vi "ATF-Connect disconnect button logic.vi"(8 "error in":errorcluster, 10 "Select type":T1, 11 "?":T2) -> (0 "error out":errorcluster, 3 "status":string)   [LabVIEW 2022 SP3]
uses:
  Controls/main case.ctl
  Controls/SeCrTs-boolean ref.ctl
  Controls/SeCrTs-EPV .ctl
  Controls/Commands to log.ctl
  UI Message handler/Message Queue/All Message Queues.ctl
  UI Message handler/Message Queue/Message Cluster.ctl
  Controls/SeCrTs-Notifier ctl.ctl
  Controls/SeCrTs-NS Data type.ctl
  Controls/ATF-Select device.ctl
  72e63059-1317-46b0-bf65-451624e866a9.vi
  5898c019-a946-4b80-818d-aafbb3f0645f.vi
  UI Message handler/Message Queue/Message Queue.lvlib
types:
  T1 = typedef "ATF-Select device.ctl" = enum16{"All", "Pump", "Storage"}
  T2 = typedef "main case.ctl" = cluster{"Bol":T3, "EPV":T4, "Covers":cluster{"cover":refnum<vi>, "Login screen cover":refnum<vi>, "cover Motor":refnum<vi>, "PPSU cover":refnum<vi>}, "Log cmd":T5, "STORAGE IP":string, "PUMP IP":string, "Storage con":bool, "Pumb con":bool, "que ref":T6, "not ref":T7, "notification":cluster{"C/NC":bool, "Start/Stop Log":bool[], "Log Name":string, "Config":cluster{"AO config":cluster{"Channel_Name":string, "Channel_Number":string, "Default_Value":dbl, "Units":string}[], "AI config":cluster{"Channel_Name":string, "Channel_Number":string, "Pre_Scale_min":dbl, "Pre_Scale_max":dbl, "Sensor_min":dbl, "Sensor_max":dbl, "Units":string}[], "DI config":cluster{"Channel_Name":string, "Channel_Number":string, "Default_Value":bool, "DI invert?":bool}[], "DO config":cluster{"Channel_Name":string, "Channel_Number":string, "Default_Value":bool, "DO invert?":bool}[], "TC config":cluster{"Channel_Name":string, "Channel_Number":string, "Pre_Scale_min":dbl, "Pre_Scale_max":dbl, "units":i32, " type":i32}[], "ACC config":cluster{"Channel_Name":string, "Channel_Number":string, "Pre_Scale_min":dbl, "Pre_Scale_max":dbl, "Terminal configuration":i32, "Sensitivity":dbl, "Sensitivity units":i32}[], "SG config":cluster{"Channel_Name":string, "Channel_Number":string, "Pre_Scale_min":dbl, "Pre_Scale_max":dbl}[], "Strain Gauge Settings":cluster{"poisson ratio":dbl, "nominal gage resistance":dbl, "gage factor":dbl}, "Bridge Settings":cluster{"voltage excitation value":dbl, "voltage excitation source":i32, "initial bridge voltage":dbl, "lead wire resistance":dbl, "strain configuration":i32}, "Sample Rate":cluster{"AI Sample Rate":dbl[], "AO Sample Rate":dbl[], "DI Sample Rate":dbl[], "TC Sample Rate":dbl[], "DO Sample Rate":dbl[], "SG Sample Rate":dbl[], "ACC Sample Rate":dbl[]}, "Drive":cluster{"Drive_Health":bool, "Drive_Frequency":u32, "Drive_Status":bool, "Drive_RPM":u32, "Drive_Direction":bool, "Acceleration state":bool, "Steady state":bool, "Deceleration state":bool, "Drive_Enable":bool, "Drive set_RPM":dbl}}, "Log min":dbl}, "Exit Drive ATF":refnum<vi>}
  T3 = typedef "SeCrTs-boolean ref.ctl" = cluster{"Connect RT":refnum<vi>, "START DAQ":refnum<vi>, "STOP DAQ":refnum<vi>, "DAQ SETTING":refnum<vi>, "START LOG":refnum<vi>, "STOP LOG":refnum<vi>, "Connect Drive ATF":refnum<vi>, "Update drive ATF":refnum<vi>, "Gate driver ATF":refnum<vi>, "Motor On ATF":refnum<vi>, "ADC reset ATF":refnum<vi>, "Gate driver ATF 2":refnum<vi>, "Motor off ATF":refnum<vi>, "MCU reset ATF":refnum<vi>, "Connect Drive Lox":refnum<vi>, "Update drive lox":refnum<vi>, "Gate driver- LOX":refnum<vi>, "Motor On lox":refnum<vi>, "Adc reset lox":refnum<vi>, "MCU Reset -LOX":refnum<vi>, "Motor Off lox":refnum<vi>, "Connect ppsu":refnum<vi>, "update ppsu":refnum<vi>, "DC on":refnum<vi>, "Alarm ack":refnum<vi>, "DC off":refnum<vi>, "Ms initialize":refnum<vi>, "Exit RT":refnum<vi>, "ABORT":refnum<vi>, "HOLD UPDATE":refnum<vi>, "Log type":refnum<vi>, "PUMP IP":refnum<vi>, "STORAGE IP":refnum<vi>}
  T4 = typedef "SeCrTs-EPV .ctl" = cluster{"F_EPV_131":refnum<vi>, "F_EPV_132":refnum<vi>, "F_EPV_136":refnum<vi>, "F_EPV_21":refnum<vi>, "F_EPV_41":refnum<vi>, "N_EPV_68":refnum<vi>, "N_EPV_ 69":refnum<vi>, "N_EPV_ 33":refnum<vi>, "F_EPV_142":refnum<vi>, "F_EPV_28":refnum<vi>, "N_EPV_203":refnum<vi>, "N_EPV_206":refnum<vi>, "F_EPV_75":refnum<vi>, "C_EPV_2":refnum<vi>, "C_EPV_7":refnum<vi>, "C_EPV_8":refnum<vi>, "C_EPV_123":refnum<vi>, "C_EPV_124":refnum<vi>, "C_EPV_127":refnum<vi>, "N_EPV_62a":refnum<vi>, "N_EPV_62b":refnum<vi>, "N_EPV_61":refnum<vi>, "G_EPV_51":refnum<vi>, "N_EPV_141":refnum<vi>, "C_EPV_803":refnum<vi>, "C_EPV_18":refnum<vi>, "C_EPV_1352":refnum<vi>, "N_EPV_202":refnum<vi>, "C_EPV_16":refnum<vi>}
  T5 = typedef "Commands to log.ctl" = cluster{"C/NC":bool, "Start/Stop Log":bool[], "Log Name":string, "Config":cluster{"AO config":cluster{"Channel_Name":string, "Channel_Number":string, "Default_Value":dbl, "Units":string}[], "AI config":cluster{"Channel_Name":string, "Channel_Number":string, "Pre_Scale_min":dbl, "Pre_Scale_max":dbl, "Sensor_min":dbl, "Sensor_max":dbl, "Units":string}[], "DI config":cluster{"Channel_Name":string, "Channel_Number":string, "Default_Value":bool, "DI invert?":bool}[], "DO config":cluster{"Channel_Name":string, "Channel_Number":string, "Default_Value":bool, "DO invert?":bool}[], "TC config":cluster{"Channel_Name":string, "Channel_Number":string, "Pre_Scale_min":dbl, "Pre_Scale_max":dbl, "units":i32, " type":i32}[], "ACC config":cluster{"Channel_Name":string, "Channel_Number":string, "Pre_Scale_min":dbl, "Pre_Scale_max":dbl, "Terminal configuration":i32, "Sensitivity":dbl, "Sensitivity units":i32}[], "SG config":cluster{"Channel_Name":string, "Channel_Number":string, "Pre_Scale_min":dbl, "Pre_Scale_max":dbl}[], "Strain Gauge Settings":cluster{"poisson ratio":dbl, "nominal gage resistance":dbl, "gage factor":dbl}, "Bridge Settings":cluster{"voltage excitation value":dbl, "voltage excitation source":i32, "initial bridge voltage":dbl, "lead wire resistance":dbl, "strain configuration":i32}, "Sample Rate":cluster{"AI Sample Rate":dbl[], "AO Sample Rate":dbl[], "DI Sample Rate":dbl[], "TC Sample Rate":dbl[], "DO Sample Rate":dbl[], "SG Sample Rate":dbl[], "ACC Sample Rate":dbl[]}}, "Log min":dbl, "Drive":cluster{"Drive_Health":bool, "Drive_Frequency":u32, "Drive_Status":bool, "Drive_RPM":u32, "Drive_Direction":bool, "Acceleration state":bool, "Steady state":bool, "Deceleration state":bool, "Drive_Enable":bool, "Drive set_RPM":dbl}, "HOLD UPDATE":bool}
  T6 = typedef "Message Queue.lvlib/All Message Queues.ctl" = cluster{"UI":refnum<queue>, "ER":refnum<queue>, "Ev":refnum<queue>, "R ER Storage":refnum<queue>, "PPSU":refnum<queue>, "R ER Pumb":refnum<queue>}
  T7 = typedef "SeCrTs-Notifier ctl.ctl" = cluster{"Storage Data":refnum<notifier>, "Pumb Data":refnum<notifier>, "Log cmd":refnum<notifier>}
  T8 = enum8{"Enabled", "Disabled", "Disabled and Grayed Out"}
  T9 = enum8{"Enabled", "Disabled", "Disabled and Grayed Out"}[]
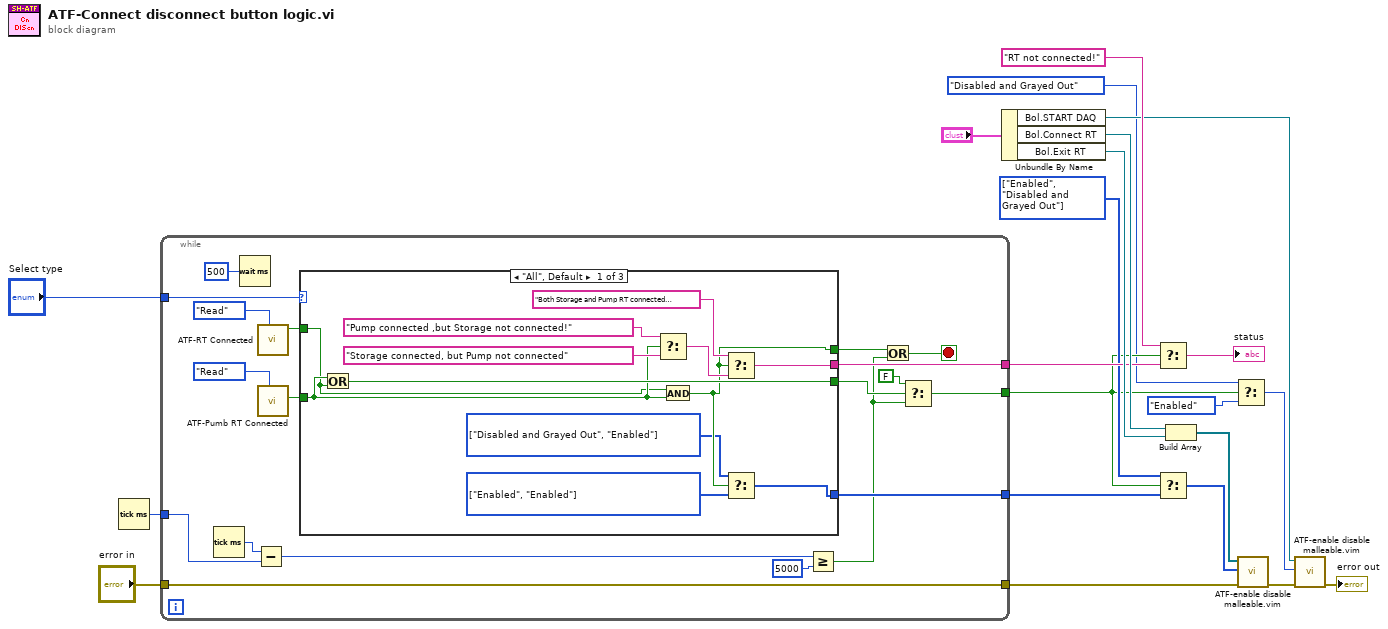
[diagram p0: block diagram]
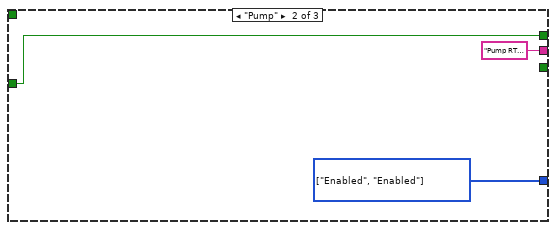
[diagram p2: hidden frame]
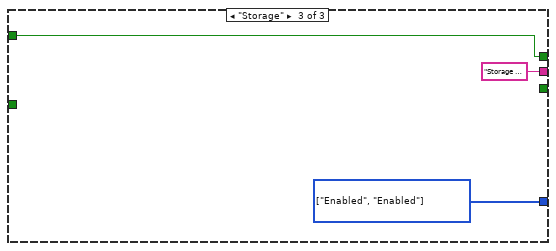
[diagram p3: hidden frame]
diagram:
  w10 = T9 [enum."Enabled", enum."Disabled and Grayed Out"] items=["Enabled", "Disabled", "Disabled and Grayed Out"] ("t")
  n1 = Tick Count (ms)() -> (millisecond timer value=w18:u32)
  n2 = while {
    tunnel: "error in" -> [w40]
    tunnel: [w40] -> w8
    tunnel: w18 -> [w38]
    tunnel: "Select type" -> [w32]
    tunnel: [w29] -> w14
    tunnel: [w28] -> w13
    tunnel: [w27] -> w4
    stop <- w30 stop-if-true
    n3 = Tick Count (ms)() -> (millisecond timer value=w39:u32)
    n4 = Wait (ms)(milliseconds to wait=u32 500) -> ()  [unwired: 1 out]
    n5 = Subtract(x=w39, y=w38) -> (x-y=w37:u32)
    n6 = call "ATF-RT Connected.vi"("Enum"=enum16{"Read", "Write"}."Read") -> ("Stoarge rt con R"=w33:bool)  [unwired: 9 in, 1 out]
    n7 = call "ATF-Pumb RT Connected.vi"("Enum"=enum16{"Read", "Write"}."Read") -> ("Pumb rt con R"=w22:bool)  [unwired: 9 in, 1 out]
    n8 = case shown="\"All\", Default" w32 {
      tunnel: w33 -> [w45 _ w58]
      tunnel: w22 -> [w46 w55 _]
      tunnel: [w44 w55 w58] -> w31
      tunnel: [w41 w54 w56] -> w29
      tunnel: [w48 "Pump RT has been connected." "Storage RT has been connected."] -> w28
      tunnel: [w47 _ _] -> w26
      frame "All", Default {
        w42 = T9 [enum."Enabled", enum."Enabled"] items=["Enabled", "Disabled", "Disabled and Grayed Out"] ("Data out")
        w43 = T9 [enum."Disabled and Grayed Out", enum."Enabled"] items=["Enabled", "Disabled", "Disabled and Grayed Out"] ("Data out")
        n9 = Or(x=w46, y=w45) -> (x .or. y?=w47:bool)
        n10 = Select(t="Pump connected ,but Storage not connected!", s=w46, f="Storage connected, but Pump not connected") -> (s? t:f=w51:string)
        n11 = And(x=w45, y=w46) -> (x .and. y?=w44:bool)
        n12 = Select(t="Both Storage and Pump RT connected Successfully.", s=w44, f=w51) -> (s? t:f=w48:string)
        n13 = Select(t=w43, s=w44, f=w42) -> (s? t:f=w41:T9)
      }
      frame "Pump" {
        w54 = T9 [enum."Enabled", enum."Enabled"] items=["Enabled", "Disabled", "Disabled and Grayed Out"] ("Data out")
      }
      frame "Storage" {
        w56 = T9 [enum."Enabled", enum."Enabled"] items=["Enabled", "Disabled", "Disabled and Grayed Out"] ("Data out")
      }
    }
    n14 = Greater Or Equal?(x=w37, y=u32 5000) -> (x >= y?=w24:bool)
    n15 = Or(x=w31, y=w24) -> (x .or. y?=w30:bool)
    n16 = Select(t=FALSE, s=w26, f=w24) -> (s? t:f=w27:bool)
  }
  n17 = Unbundle By Name("?") -> ("Bol.START DAQ"=w5:refnum<vi>, "Bol.Connect RT"=w17:refnum<vi>, "Bol.Exit RT"=w16:refnum<vi>)
  n18 = Select(t="RT not connected!", s=w4, f=w13) -> (s? t:f=→"status":string)
  n19 = Select(t=w10, s=w4, f=w14) -> (s? t:f=w9:T9)
  n20 = Build Array(w17, w16) -> (w15:refnum<vi>[])
  n21 = Select(t=T8."Disabled and Grayed Out" ("Disabled"), s=w4, f=T8."Enabled" ("Disabled")) -> (s? t:f=w1:T8)
  n22 = call "ATF-enable disable malleable.vim"("error in"=w8, "Data"=w9, "Ref in"=w15) -> ("error out"=w7:errorcluster)  [unwired: 7 in, 1 out]
  n23 = call "ATF-enable disable malleable.vim"("error in"=w7, "Data"=w1, "Ref in"=w5) -> ("error out"=→"error out":errorcluster)  [unwired: 7 in, 1 out]
